vi "GetChannels.vi"(7 "ModuleID":i32, 8 "error in (no error)":errorcluster, 11 "ScopePluginsBase in":refnum<class "ScopePluginsBase.lvclass">) -> (0 "error out":errorcluster, 3 "ScopePluginsBase out":refnum<class "ScopePluginsBase.lvclass">)   [LabVIEW 2018, in "ScopePlugins.lvlib" / "ScopePluginsBase.lvclass"]
uses:
  ScopePluginsBase.lvclass
  ScopePluginsBase.lvclass/ScopePluginsBase.ctl
  Accessors/Read Channels.vi
  ScopePlugins.lvlib
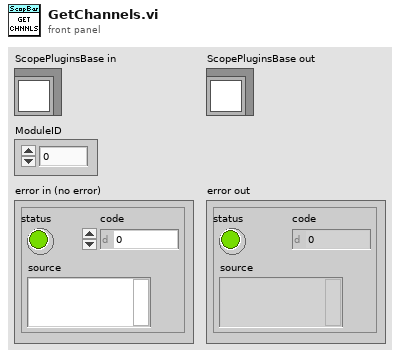
[diagram p1: front panel]
types:
  T1 = typedef "ScopePlugins.lvlib/ScopePluginsBase.lvclass/ChannelSetting(s).ctl" = cluster{"Number of Channels":i32, "Channel(s)":cluster{"Enabled":bool, "Instrument Handle":string, "Channel Name":string, "Maximum Input Frequency":dbl, "Verticle Settings":cluster{"Vertical Range":dbl, "Vertical Offset":dbl, "Probe Attenuation":dbl, "Vertical Coupling":i32}, "Connected":bool, "Input Impedance":dbl, "IO Type Instrument Handle":refnum<k15>}[]}
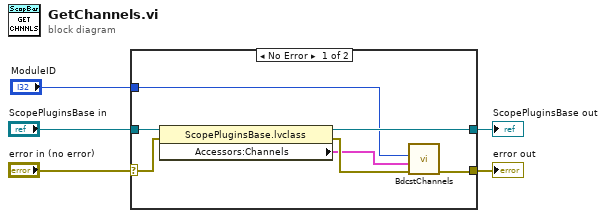
[diagram p0: block diagram]
diagram:
  n1 = case shown="No Error" "error in (no error)" {
    selector: "error in (no error)" -> [w8 w14]
    tunnel: [w9 w14] -> w4
    tunnel: [w11 w13] -> w2
    tunnel: "ScopePluginsBase in" -> [w12 w13]
    tunnel: "ModuleID" -> [w10 _]
    frame No Error {
      n2 = property class="ScopePluginsBase.lvclass"(reference=w12, error in=w8) -> (reference out=w11:refnum<class "ScopePluginsBase.lvclass">, error out=w7:errorcluster, "Accessors:Channels"=w6:T1)
      n3 = call "BdcstChannels.vi"("error in (no error)"=w7, "Channels"=w6, "ModuleID"=w10) -> ("error out"=w9:errorcluster)  [unwired: 8 in]
    }
    frame Error {
    }
  }
  "error out" <- w4
  "ScopePluginsBase out" <- w2
